vi "Quickbooks Online OAuth Test.vi"() -> ()   [LabVIEW 2013]
uses:
  Oauth2.QBO/QBO Access Scopes.ctl
  OauthClient/OAuthClient.lvclass
  Oauth2.QBO/Oauth2.QBO.lvclass
  Oauth2/Oauth2.lvclass/Oauth2.ctl
  Oauth2/Read RefreshToken.vi
  Oauth2/Read ExpiresIn.vi
  Oauth2/Read Redirect URI.vi
  OAuthToken/Retrieve Element.vi
  Oauth2/Oauth2.lvclass
  <vilib>/LabVIEW Open Source Project/OpenURI/uri/URI.lvclass
  <vilib>/httpClient/LabVIEWHTTPClient.lvlib
panel:
  in  "API Server":T1(ring)
  in  "QBO Access Scope":T2={"com.intuit.quickbooks.accounting\t"=TRUE, "com.intuit.quickbooks.payment\t"=FALSE, "openid\t"=FALSE}
  out "REST API Error":errorcluster
  out "HTTP Response Headers":string
  out "Accounts":string
  out "Harvest Access Token":string
  out "Refresh Token":string
  out "Expires In":u32
  out "Redirect URI":string
  out "Oauth Error":errorcluster
  in  "Query Company Info":bool
  in  "Refresh":bool
  in  "Authorize":bool
  in  "Client Secret":string
  in  "Client ID":string
  # "Quickbooks Online Application API Access Example"
  # "G Open Source Project for LabVIEW\nhttps://github.com/LabVIEW-Open-Source/Oauth2"
  # "1- Get a Client ID and Client Secret from the application's admin. \n\n          * To access your own account, log into your site, create an application and set the access scope. \n          * This Oauth2.0 API uses the following redirect URL: http://localhost:58888/Oauth2/Redirect\n          * Record the client ID and client secret and fill in the fields below."
  # "3- Get an Access Token. You will be redirected your QBO App's Authorization Server URI\n              * To authorize access, click on the \"Authorize App\" button.\n\n4- Once you have authenticated yourself, you will receive an access token.\n              * Use the \"Refresh Token\" button to request a fresh token\n                       OR\n              * Use the Access Token to query the QBO API"
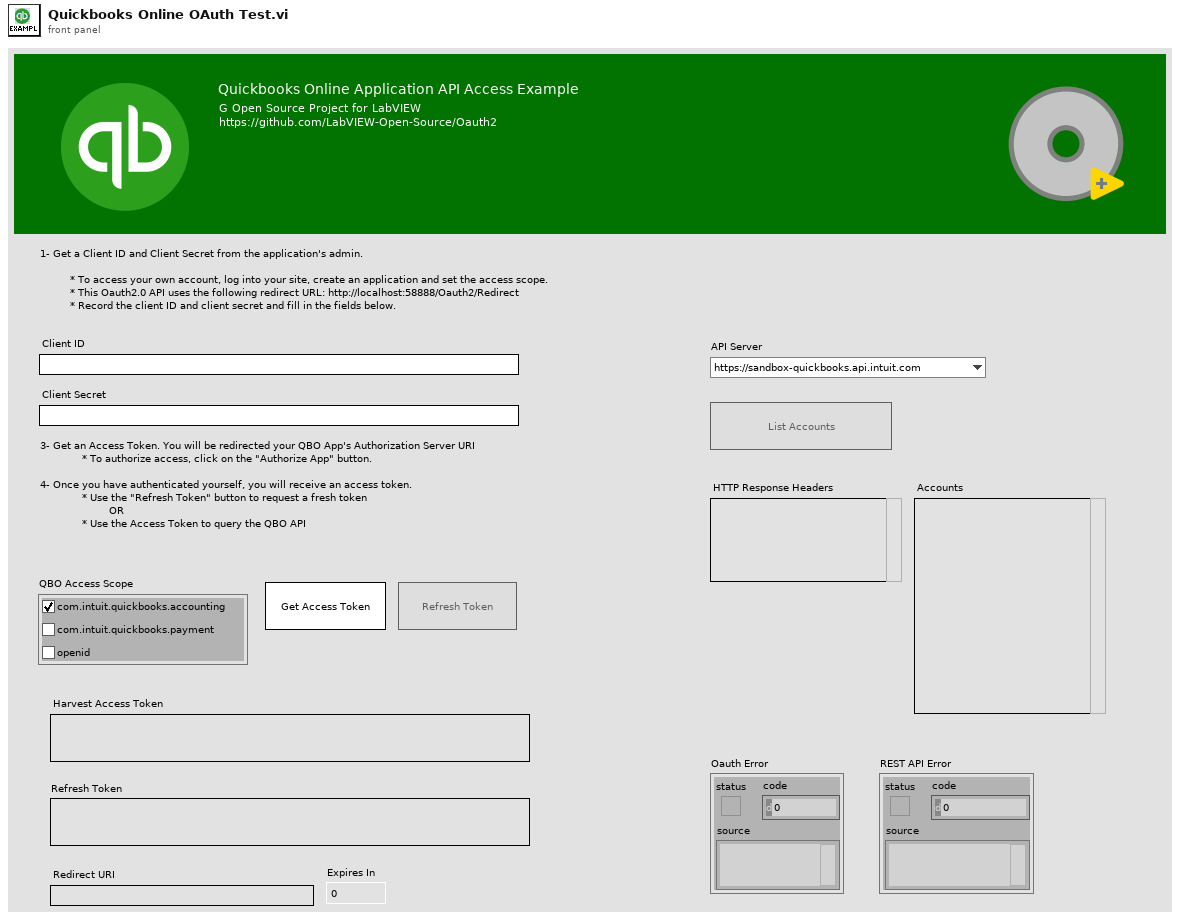
[diagram p1: front panel]
types:
  T1 = enum16{"https://sandbox-quickbooks.api.intuit.com", "https://quickbooks.api.intuit.com"}
  T2 = typedef "Oauth2.QBO.lvclass/QBO Access Scopes.ctl" = cluster{"com.intuit.quickbooks.accounting\t":bool, "com.intuit.quickbooks.payment\t":bool, "openid\t":bool}
  T3 = cluster{"Oauth2":refnum<class "Oauth2.QBO.lvclass">, "Base API":string}
  T4 = enum8{"Enabled", "Disabled", "Disabled and Grayed Out"}
  T5 = typedef "LabVIEWHTTPClient.lvlib/ClientHandle.ctl" = refnum<k1>
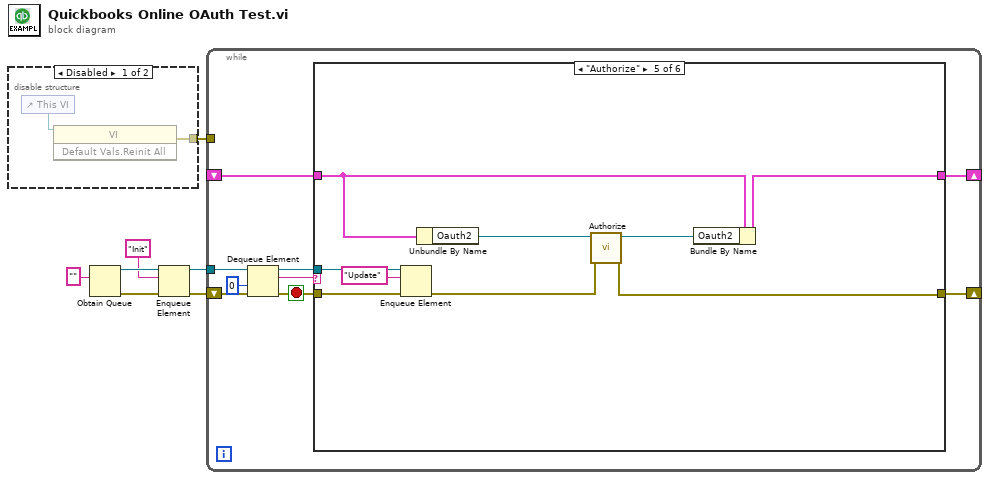
[diagram p0: block diagram]
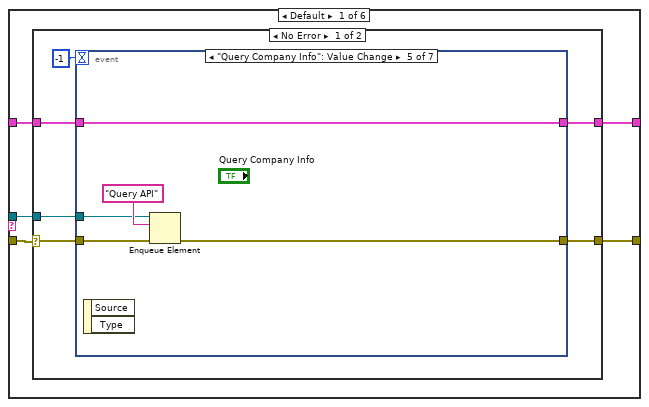
[diagram p3: hidden frame]
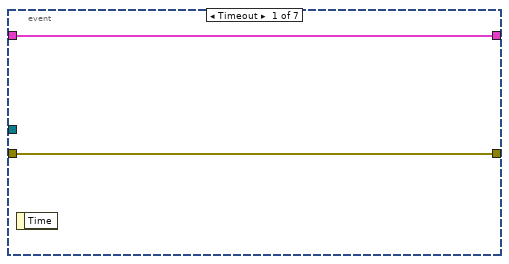
[diagram p4: hidden frame]
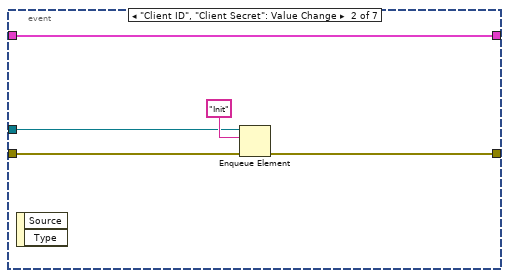
[diagram p5: hidden frame]
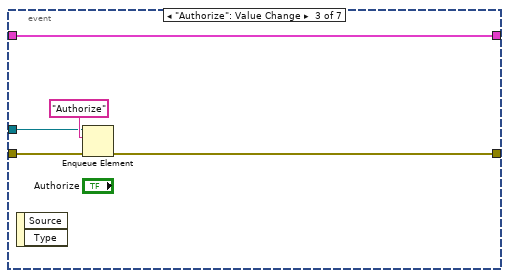
[diagram p6: hidden frame]
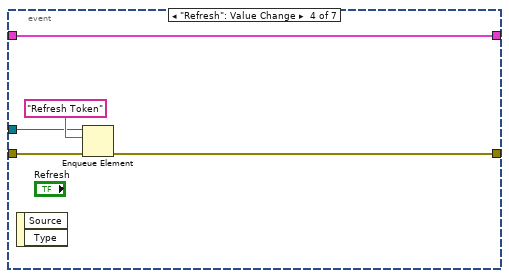
[diagram p7: hidden frame]
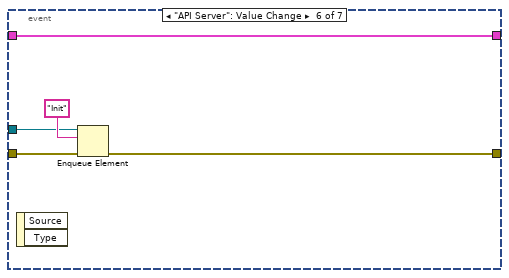
[diagram p8: hidden frame]
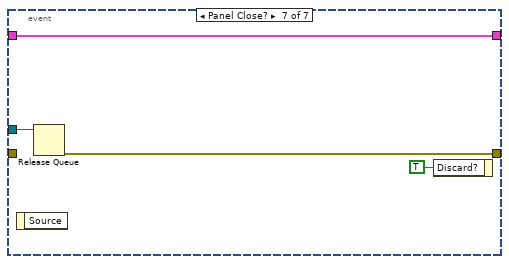
[diagram p9: hidden frame]
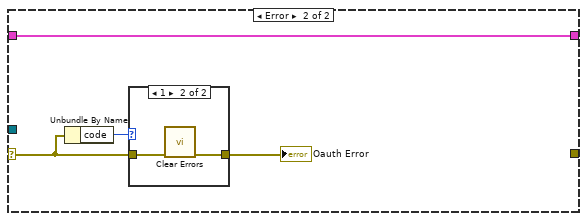
[diagram p10: hidden frame]
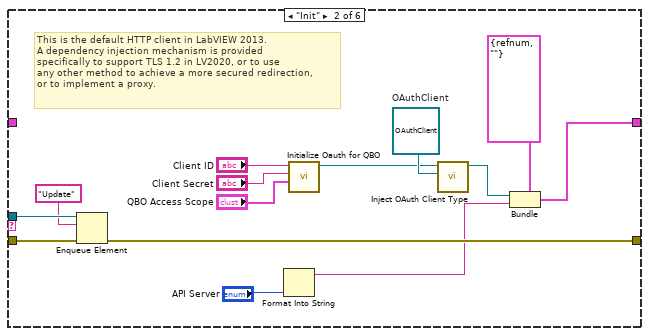
[diagram p12: hidden frame]
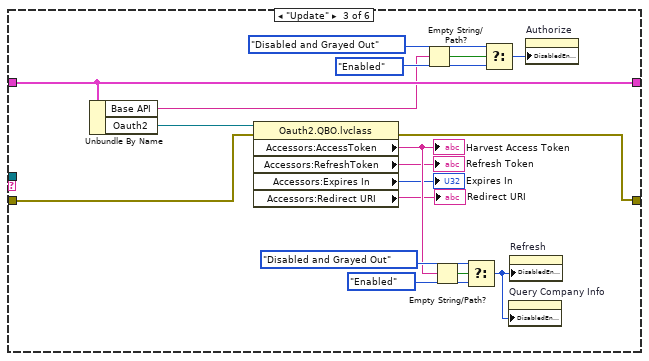
[diagram p13: hidden frame]
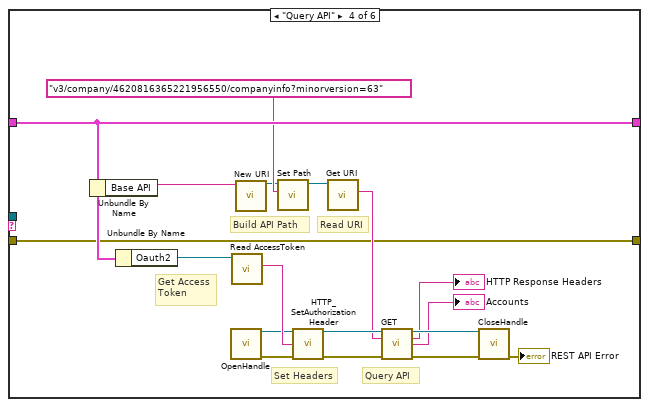
[diagram p14: hidden frame]
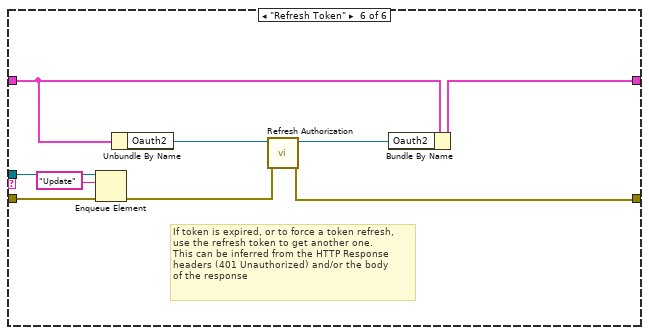
[diagram p15: hidden frame]
diagram:
  n1 = disable-structure shown="Disabled" {
    disable-tunnel: [w8 _] -> w1
    frame Disabled {
      n2 = control-ref of="This VI"() -> (w9:refnum<vi>)
      n3 = invoke class="VI" method="Default Vals.Reinit All"(reference=w9) -> (error out=w8:errorcluster)  [unwired: 2 in, 2 out]
    }
    frame Enabled {
    }
  }
  n4 = Obtain Queue(element data type="") -> (queue out=w4:refnum<queue>, error out=w6:errorcluster)  [unwired: 4 in, 1 out]
  n5 = Enqueue Element(queue=w4, element="Init", error in (no error)=w6) -> (queue out=w3:refnum<queue>, error out=w5:errorcluster)  [unwired: 1 in, 1 out]
  n6 = while {
    tunnel: w3 -> [w18]
    shift-right: [w13] -> _
    shift-left: _ -> [w12]
    shift-right: [w10] -> _
    shift-left: w5 -> [w14]
    tunnel: w1 -> [_]
    stop <- w11 stop-if-true
    n7 = Dequeue Element(queue=w18, timeout in ms (-1)=0, error in (no error)=w14) -> (queue out=w15:refnum<queue>, element=w16:string, error out=w11:errorcluster)  [unwired: 1 out]
    n8 = case shown="\"Authorize\"" w16 {
      tunnel: w15 -> [w23 w80 _ _ w119 w131]
      tunnel: [w22 w81 w98 w113 w121 w133] -> w13
      tunnel: w12 -> [w21 _ w98 w113 w122 w134]
      tunnel: w11 -> [w20 w77 w88 w101 w118 w130]
      tunnel: [w19 w78 w87 w101 w124 w126] -> w10
      frame Default {
        n9 = case shown="No Error" w20 {
          selector: w20 -> [w24 w63]
          tunnel: w23 -> [w28 _]
          tunnel: [w27 w64] -> w22
          tunnel: w21 -> [w26 w64]
          tunnel: [w25 _] -> w19
          frame No Error {
            n10 = event shown="[4] \"Query Company Info\": Value Change" {
              selector: _ -> [_ _ _ _ _ _ _]
              dyn-events: _ -> [_ _ _ _ _ _ _]
              timeout: -1 -> [_ _ _ _ _ _ _]
              tunnel: w28 -> [_ w34 w40 w45 w50 w55 w60]
              tunnel: [w31 w36 w38 w43 w48 w53 w58] -> w27
              tunnel: w26 -> [w31 w36 w38 w43 w48 w53 w58]
              tunnel: [w30 w32 w37 w42 w47 w52 w57] -> w25
              tunnel: w24 -> [w30 w33 w39 w44 w49 w54 _]
              event Timeout {
                n11 = event-data() -> ()  [unwired: 1 in, 1 out]
              }
              event "Client ID", "Client Secret": Value Change {
                n12 = event-data() -> ()  [unwired: 1 in, 2 out]
                n13 = Enqueue Element(queue=w34, element="Init", error in (no error)=w33) -> (error out=w32:errorcluster)  [unwired: 1 in, 2 out]
              }
              event "Authorize": Value Change {
                n14 = event-data() -> ()  [unwired: 1 in, 2 out]
                n15 = Enqueue Element(queue=w40, element="Authorize", error in (no error)=w39) -> (error out=w37:errorcluster)  [unwired: 1 in, 2 out]
              }
              event "Refresh": Value Change {
                n16 = event-data() -> ()  [unwired: 1 in, 2 out]
                n17 = Enqueue Element(queue=w45, element="Refresh Token", error in (no error)=w44) -> (error out=w42:errorcluster)  [unwired: 1 in, 2 out]
              }
              event "Query Company Info": Value Change {
                n18 = event-data() -> ()  [unwired: 1 in, 2 out]
                n19 = Enqueue Element(queue=w50, element="Query API", error in (no error)=w49) -> (error out=w47:errorcluster)  [unwired: 1 in, 2 out]
              }
              event "API Server": Value Change {
                n20 = event-data() -> ()  [unwired: 1 in, 2 out]
                n21 = Enqueue Element(queue=w55, element="Init", error in (no error)=w54) -> (error out=w52:errorcluster)  [unwired: 1 in, 2 out]
              }
              event Panel Close? {
                n22 = event-data() -> ()  [unwired: 1 in, 1 out]
                n23 = Release Queue(queue=w60) -> (error out=w57:errorcluster)  [unwired: 2 in, 2 out]
                n24 = event-data("Discard?"=TRUE) -> ()  [unwired: 1 in, 1 out]
              }
            }
          }
          frame Error {
            n25 = Unbundle By Name(w63) -> ("code"=w61:i32)
            n26 = case shown="1" w61 {
              tunnel: w63 -> [w65 w67]
              tunnel: [w65 w66] -> w62
              frame Default {
              }
              frame 1 {
                n27 = call <vilib>:"Clear Errors.vi"("error in (no error)"=w67) -> ("error out"=w66:errorcluster)  [unwired: 6 in]
              }
            }
            "Oauth Error" <- w62
          }
        }
      }
      frame "Init" {
        w76 = refnum<class "OAuthClient.lvclass"> refnum  # OAuthClient
        # "This is the default HTTP client in LabVIEW 2013.\nA dependency injection mechanism is provided\nspecifically to support TLS 1.2 in LV2020, or to use\nany other method to achieve a more secured redirection, \nor to implement a proxy."
        n28 = Enqueue Element(queue=w80, element="Update", error in (no error)=w77) -> (error out=w78:errorcluster)  [unwired: 1 in, 2 out]
        n29 = Format Into String("API Server") -> (resulting string=w69:string)  [unwired: 3 in, 1 out]
        n30 = call "Initialize Oauth for QBO.vi"("QBO Access Scope"="QBO Access Scope", "Client Secret"="Client Secret", "Client ID"="Client ID") -> ("Oauth2.QBO"=w72:refnum<class "Oauth2.QBO.lvclass">)  [unwired: 7 in, 1 out]
        n31 = call "Inject OAuth Client Type.vi"("OAuthClient"=w76, "Oauth2 in"=w72) -> ("Oauth2"=w75:refnum<class "Oauth2.QBO.lvclass">)  [unwired: 9 in]
        n32 = Bundle(cluster=T3 {"Oauth2"=refnum, "Base API"=""}, "Oauth2"=w75, "Base API"=w69) -> (w81:T3)
      }
      frame "Update" {
        n33 = Unbundle By Name(w98) -> ("Base API"=w92:string, "Oauth2"=w93:refnum<class "Oauth2.QBO.lvclass">)
        n34 = property class="Oauth2.QBO.lvclass"(reference=w93, error in=w88) -> (error out=w87:errorcluster, "Accessors:AccessToken"=w86:string, "Accessors:RefreshToken"=→"Refresh Token":string, "Accessors:Expires In"=→"Expires In":u32, "Accessors:Redirect URI"=→"Redirect URI":string)  [unwired: 1 out]
        "Harvest Access Token" <- w86
        n35 = Empty String/Path?(string/path=w92) -> (empty?=w95:bool)
        n36 = Empty String/Path?(string/path=w86) -> (empty?=w91:bool)
        n37 = Select(t=T4."Disabled and Grayed Out" ("Disabled"), s=w91, f=T4."Enabled" ("Disabled")) -> (s? t:f=w82:T4)
        n38 = Select(t=T4."Disabled and Grayed Out" ("Disabled"), s=w95, f=T4."Enabled" ("Disabled")) -> (s? t:f=w94:T4)
        n39 = property on="Query Company Info" class="Bool"("DisabledEnum"=w82) -> ()  [unwired: 2 in, 2 out]
        n40 = property on="Refresh" class="Bool"("DisabledEnum"=w82) -> ()  [unwired: 2 in, 2 out]
        n41 = property on="Authorize" class="Bool"("DisabledEnum"=w94) -> ()  [unwired: 2 in, 2 out]
      }
      frame "Query API" {
        # "Query API"
        # "Set Headers"
        # "Get Access\nToken"
        # "Read URI"
        # "Build API Path"
        n42 = Unbundle By Name(w113) -> ("Base API"=w109:string)
        n43 = Unbundle By Name(w113) -> ("Oauth2"=w114:refnum<class "Oauth2.QBO.lvclass">)
        n44 = call <vilib>:"OpenHandle.vi"() -> ("client handle out"=w115:T5, "error out"=w106:errorcluster)  [unwired: 14 in]
        n45 = call "Read AccessToken.vi"("Oauth2 in"=w114) -> ("Access Token"=w116:string)  [unwired: 8 in, 2 out]
        n46 = call <vilib>:"New URI.vi"("URI"=w109) -> ("URI"=w110:refnum<class "URI.lvclass">)  [unwired: 9 in, 1 out]
        n47 = call <vilib>:"Set Path.vi"("path"="v3/company/4620816365221956550/companyinfo?minorversion=63", "URI in"=w110) -> ("URI out"=w112:refnum<class "URI.lvclass">)  [unwired: 8 in, 1 out]
        n48 = call "HTTP_SetAuthorizationHeader.vi"("Client Handle"=w115, "Access Token"=w116, "error in (no error)"=w106) -> ("client handle dup"=w108:T5, "error out"=w105:errorcluster)  [unwired: 11 in]
        n49 = call <vilib>:"Get URI.vi"("URI in"=w112) -> ("URI String"=w107:string)  [unwired: 8 in, 2 out]
        n50 = call <vilib>:"GET.vi"("client handle"=w108, "url"=w107, "error in (no error)"=w105) -> ("client handle out"=w104:T5, "headers"=→"HTTP Response Headers":string, "body"=→"Accounts":string, "error out"=w103:errorcluster)  [unwired: 9 in]
        n51 = call <vilib>:"CloseHandle.vi"("client handle"=w104, "error in (no error)"=w103) -> ("error out"=→"REST API Error":errorcluster)  [unwired: 13 in]
      }
      frame "Authorize" {
        n52 = Enqueue Element(queue=w119, element="Update", error in (no error)=w118) -> (error out=w117:errorcluster)  [unwired: 1 in, 2 out]
        n53 = Unbundle By Name(w122) -> ("Oauth2"=w125:refnum<class "Oauth2.QBO.lvclass">)
        n54 = call "Authorize.vi"("error in (no error)"=w117, "Oauth2 in"=w125) -> ("error out"=w124:errorcluster, "Oauth2 out"=w123:refnum<class "Oauth2.QBO.lvclass">)  [unwired: 7 in, 1 out]
        n55 = Bundle By Name(cluster=w122, "Oauth2"=w123) -> (w121:T3)
      }
      frame "Refresh Token" {
        # "If token is expired, or to force a token refresh, \nuse the refresh token to get another one.\nThis can be inferred from the HTTP Response\nheaders (401 Unauthorized) and/or the body\nof the response"
        n56 = Enqueue Element(queue=w131, element="Update", error in (no error)=w130) -> (error out=w127:errorcluster)  [unwired: 1 in, 2 out]
        n57 = Unbundle By Name(w134) -> ("Oauth2"=w129:refnum<class "Oauth2.QBO.lvclass">)
        n58 = call "Refresh Authorization.vi"("error in (no error)"=w127, "Oauth2 in"=w129) -> ("error out"=w126:errorcluster, "Oauth2 out"=w128:refnum<class "Oauth2.QBO.lvclass">)  [unwired: 7 in, 1 out]
        n59 = Bundle By Name(cluster=w134, "Oauth2"=w128) -> (w133:T3)
      }
    }
  }
